vi "Test.vi"() -> (4 "Encoders Working\n(backwards)":bool, 6 "Encoders Working\n(forwards)":bool, 8 "Event Passed In Correctly":bool, 10 "LIDAR Gets Data":bool, 15 "Gyro Angle Correct 2":bool)   [LabVIEW 2017]
uses:
  Globals/Gyro.vi
  state-manager/Event.ctl
panel:
  out "Gyro Bias":dbl
  out "Camera Error":errorcluster
  out "Gyro Error":errorcluster
  out "LIDAR Error":errorcluster
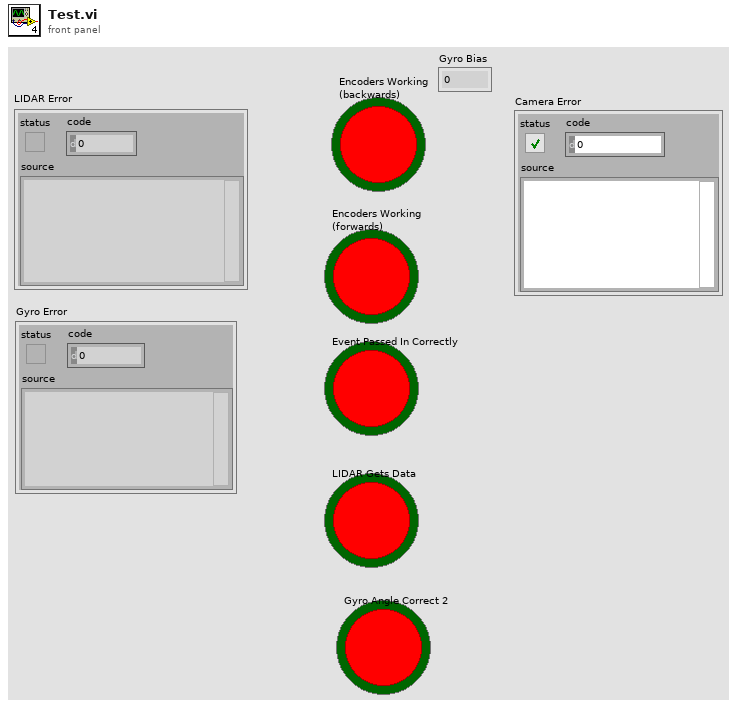
[diagram p1: front panel]
types:
  T1 = typedef "I2C.lvlib/I2C Reference.ctl" = cluster{"myRIO Reference":T2, "I2C Channels Enum":T6, "I2C Configuration":T7}
  T2 = typedef "myRIO Generic Hardware Reference.ctl" = cluster{"myRIO Model":T3, "myRIO Hardware Reference":T4}
  T3 = typedef "Hardware Version Enum.ctl" = enum16{"Unknown", "myRIO-1900", "myRIO-1950", "roboRIO", "NI ELVIS RIO CM"}
  T4 = typedef "myRIO v1.0 Reference.ctl" = cluster{"Generic FPGA Reference":T5, "Allow multiple opens":bool}
  T5 = typedef "Generic FPGA Reference.ctl" = refnum<k20>
  T6 = typedef "I2C Channels Enum.ctl" = enum16{"Not Connected", "A/I2C", "B/I2C", "I2C/I2C"}
  T7 = typedef "I2C.lvlib/I2C Configuration.ctl" = cluster{"I2C Transfer Rate":T8}
  T8 = typedef "I2C.lvlib/I2C Transfer Rate.ctl" = enum16{"Standard mode (100 kbps)", "Fast mode (400 kbps)"}
  T9 = typedef "Event.ctl" = enum16{"None", "Zig Zag Finished", "Start Obstacle Avoidance", "Start Button Pressed", "Black & Yellow Tape Touched", "Black & Yellow Tape Passed", "Green Tape Crossed", "Red Tape Touched", "Rough Terrain Touched", "Black Tape Crossed", "Tape Edge Too Close", "Wall Too Close", "Rough Terrain Passed", "Ramp Passed", "Stop Button Pressed", "Recentered", "End Zone Wait Timed Out"}
  T10 = typedef "IMAQdx.ctl" = refnum<k21>
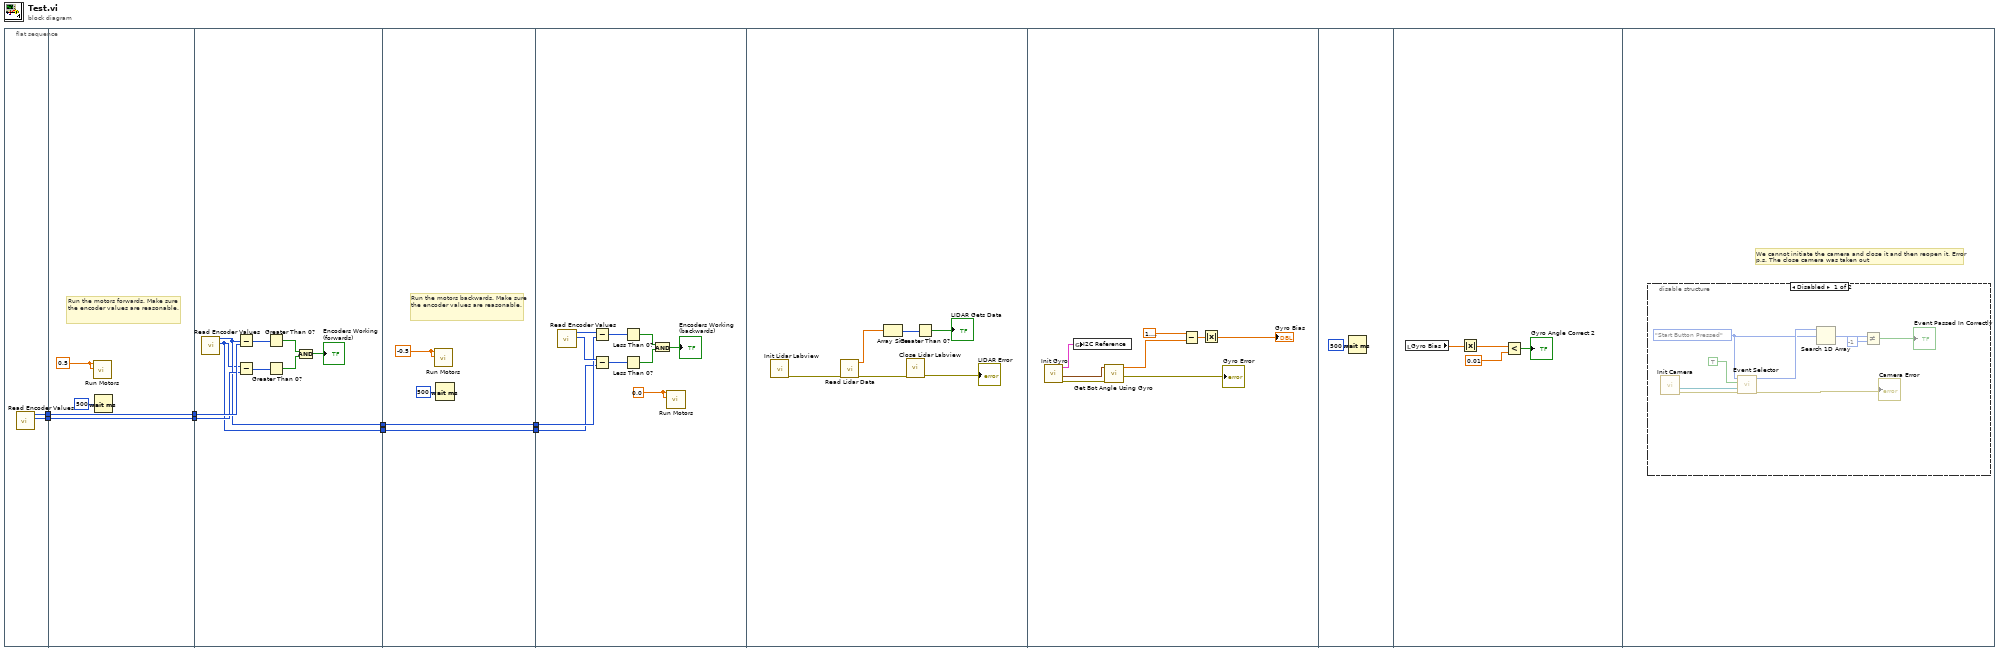
[diagram p0: block diagram]
diagram:
  n1 = flat-sequence {
    tunnel: [w10] -> w8
    tunnel: [w9] -> w7
    tunnel: w8 -> [w12]
    tunnel: w7 -> [w11]
    tunnel: [w12] -> w6
    tunnel: [w11] -> w5
    tunnel: w6 -> [w23]
    tunnel: w5 -> [w22]
    tunnel: [w16] -> w4
    tunnel: [w15] -> w3
    tunnel: w4 -> [w25]
    tunnel: w3 -> [w24]
    tunnel: [w25] -> w2
    tunnel: [w24] -> w1
    tunnel: w2 -> [w29]
    tunnel: w1 -> [w28]
    frame #0 {
      n2 = call "Read Encoder Values.vi"() -> ("Right Value"=w9:i32, "Left  Value"=w10:i32)  [unwired: 10 in]
    }
    frame #1 {
      w14 = 0.5 ("Left motor speed (-1..1)")
      # "Run the motors forwards. Make sure the encoder values are reasonable."
      n3 = call "Run Motors.vi"("Right motor side (-1..1)"=w14, "Left motor speed (-1..1)"=w14) -> ()  [unwired: 10 in]
      n4 = Wait (ms)(milliseconds to wait=u32 500) -> ()  [unwired: 1 out]
    }
    frame #2 {
      n5 = call "Read Encoder Values.vi"() -> ("Right Value"=w15:i32, "Left  Value"=w16:i32)  [unwired: 10 in]
      n6 = Subtract(x=w16, y=w23) -> (x-y=w21:i32)
      n7 = Subtract(x=w15, y=w22) -> (x-y=w20:i32)
      n8 = Greater Than 0?(x=w21) -> (x > 0?=w19:bool)
      n9 = Greater Than 0?(x=w20) -> (x > 0?=w18:bool)
      n10 = And(x=w19, y=w18) -> (x .and. y?=→"Encoders Working\n(forwards)":bool)
    }
    frame #3 {
      w26 = -0.5 ("Left motor speed (-1..1)")
      # "Run the motors backwards. Make sure the encoder values are reasonable."
      n11 = call "Run Motors.vi"("Right motor side (-1..1)"=w26, "Left motor speed (-1..1)"=w26) -> ()  [unwired: 10 in]
      n12 = Wait (ms)(milliseconds to wait=u32 500) -> ()  [unwired: 1 out]
    }
    frame #4 {
      w30 = 0.0 ("Left motor speed (-1..1)")
      n13 = call "Read Encoder Values.vi"() -> ("Right Value"=w36:i32, "Left  Value"=w37:i32)  [unwired: 10 in]
      n14 = Subtract(x=w37, y=w29) -> (x-y=w35:i32)
      n15 = Subtract(x=w36, y=w28) -> (x-y=w34:i32)
      n16 = Less Than 0?(x=w35) -> (x < 0?=w33:bool)
      n17 = Less Than 0?(x=w34) -> (x < 0?=w32:bool)
      n18 = And(x=w33, y=w32) -> (x .and. y?=→"Encoders Working\n(backwards)":bool)
      n19 = call "Run Motors.vi"("Right motor side (-1..1)"=w30, "Left motor speed (-1..1)"=w30) -> ()  [unwired: 10 in]
    }
    frame #5 {
      n20 = call "Init Lidar Labview.vi"() -> ("error out"=w43:errorcluster)  [unwired: 11 in]
      n21 = call "Read Lidar Data.vi"("error in (no error)"=w43) -> ("error out"=w42:errorcluster, "Magnitude"=w41:dbl[])  [unwired: 8 in, 1 out]
      n22 = Array Size(array=w41) -> (size(s)=w40:i32)
      n23 = call "Close Lidar Labview.vi"("error in (no error)"=w42) -> ("error out"=→"LIDAR Error":errorcluster)  [unwired: 10 in]
      n24 = Greater Than 0?(x=w40) -> (x > 0?=→"LIDAR Gets Data":bool)
    }
    frame #6 {
      n25 = call "Init Gyro.vi"() -> ("error out"=w50:errorcluster, "Gyro Bias"=w48:cluster{"X":dbl, "Y":dbl, "Z":dbl}, "I2C Ref Out"=w51:T1)  [unwired: 9 in]
      n26 = global write "Gyro.vi" "I2C Reference"(w51) -> ()
      n27 = call "Get Bot Angle Using Gyro.vi"("error in (no error)"=w50, "Gyro bias"=w48) -> ("error out"=→"Gyro Error":errorcluster, "Z Rotation (rads)"=w47:dbl)  [unwired: 6 in, 2 out]
      n28 = Subtract(x=1.5707963267948966, y=w47) -> (x-y=w45:dbl)
      n29 = Absolute Value(x=w45) -> (abs(x)=→"Gyro Bias":dbl)
    }
    frame #7 {
      n30 = Wait (ms)(milliseconds to wait=u32 500) -> ()  [unwired: 1 out]
    }
    frame #8 {
      n31 = local read "Gyro Bias"() -> (w53:dbl)
      n32 = Absolute Value(x=w53) -> (abs(x)=w54:dbl)
      n33 = Less?(x=w54, y=0.01) -> (x < y?=→"Gyro Angle Correct 2":bool)
    }
    frame #9 {
      # "We cannot initiate the camera and close it and then reopen it. Error\np.s. The close camera was taken out"
      n34 = disable-structure shown="Disabled" {
        frame Disabled {
          w58 = Event."Start Button Pressed" ("Manual Pass In Event")
          n35 = call "Init Camera.vi"() -> ("error out"=w65:errorcluster, "session out"=w64:T10)  [unwired: 9 in]
          n36 = call "Event Selector.vi"("Error In"=w65, "Session In"=w64, "Pass In Event"=TRUE, "Manual Pass In Event"=w58) -> ("Error Out"=→"Camera Error":errorcluster, "Event Queue"=w59:T9[])  [unwired: 5 in, 1 out]
          n37 = Search 1D Array(1D array=w59, element=w58) -> (index of element=w62:i32)  [unwired: 1 in]
          n38 = Not Equal?(x=w62, y=-1) -> (x != y?=→"Event Passed In Correctly":bool)
        }
        frame Enabled {
        }
      }
    }
  }
